vi "endVolume.vi"(8 "error in (no error)":errorcluster, 9 "com queue":refnum<queue>, 10 "scan info":T2, 11 "reader status in":T1) -> (0 "error out":errorcluster, 1 "com queue out":refnum<queue>, 3 "reader status out":T1)   [LabVIEW 2010]
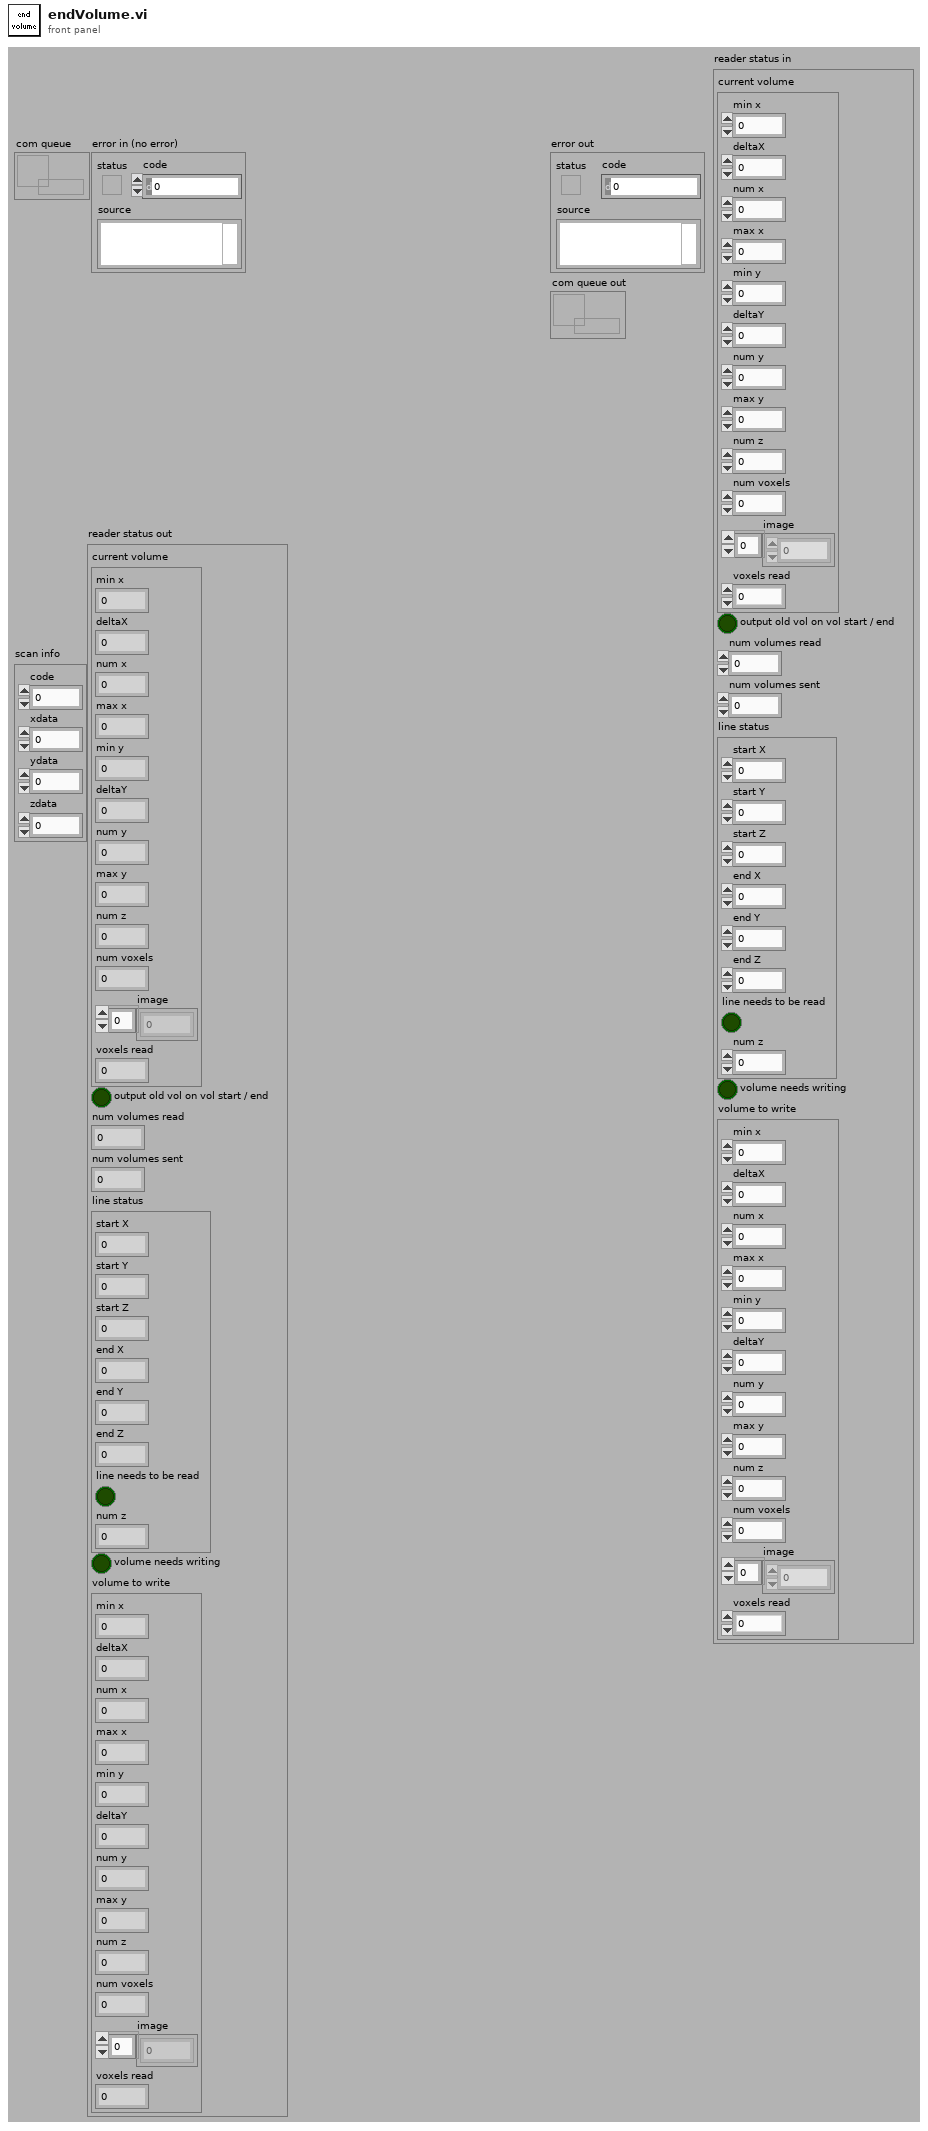
[diagram p1: front panel]
types:
  T1 = cluster{"current volume":cluster{"min x":i16, "deltaX":dbl, "num x":u32, "max x":i16, "min y":i16, "deltaY":dbl, "num y":u32, "max y":i16, "num z":u32, "num voxels":u32, "image":u32[], "voxels read":u32}, "output old vol on vol start / end":bool, "num volumes read":u32, "num volumes sent":u32, "line status":cluster{"start X":i16, "start Y":i16, "start Z":i16, "end X":i16, "end Y":i16, "end Z":i16, "line needs to be read":bool, "num z":u8}, "volume needs writing":bool, "volume to write":cluster{"min x":i16, "deltaX":dbl, "num x":u32, "max x":i16, "min y":i16, "deltaY":dbl, "num y":u32, "max y":i16, "num z":u32, "num voxels":u32, "image":u32[], "voxels read":u32}}
  T2 = cluster{"code":i32, "xdata":i32, "ydata":i32, "zdata":i32}
  T3 = enum16{"NONE", "VOLUME_START", "LINE_START", "LINE_END", "VOLUME_END"}
  T4 = cluster{"min x":i16, "deltaX":dbl, "num x":u32, "max x":i16, "min y":i16, "deltaY":dbl, "num y":u32, "max y":i16, "num z":u32, "num voxels":u32, "image":u32[], "voxels read":u32}
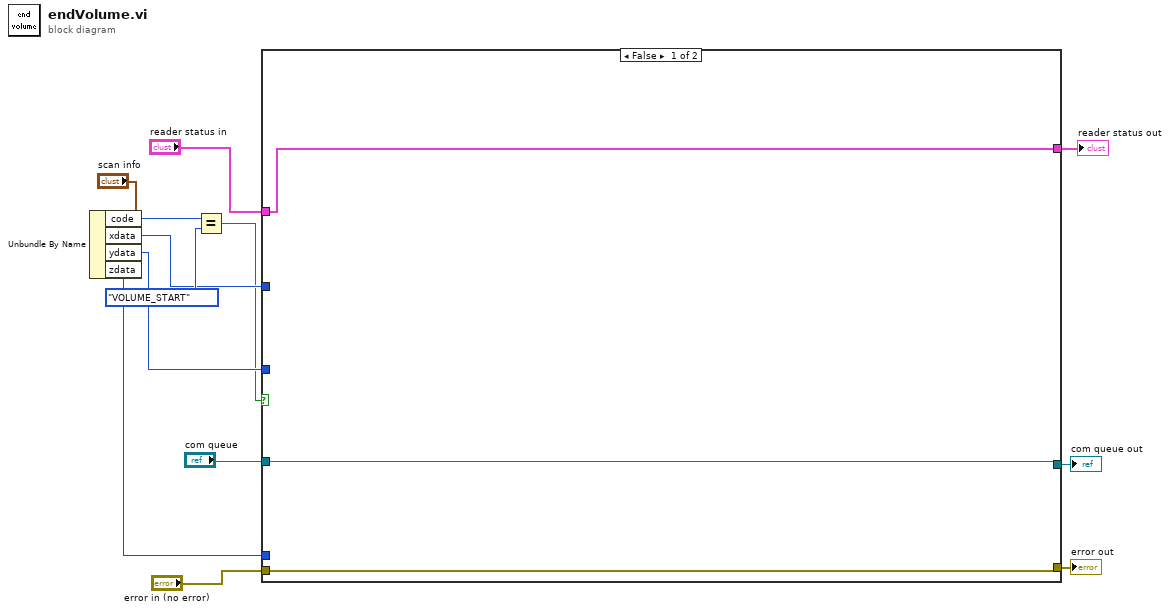
[diagram p0: block diagram]
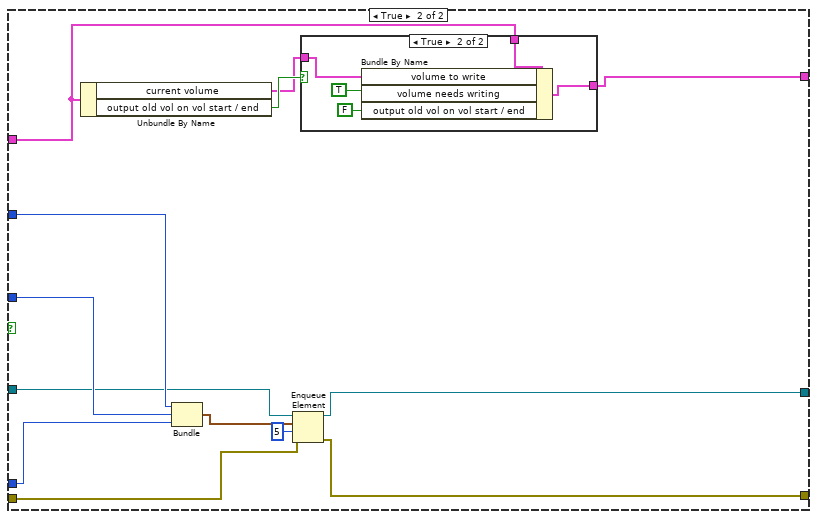
[diagram p2: hidden frame]
diagram:
  n1 = Unbundle By Name("scan info") -> ("code"=w12:i32, "xdata"=w10:i32, "ydata"=w9:i32, "zdata"=w8:i32)
  n2 = Equal?(x=w12, y=T3."VOLUME_START" ("message")) -> (x = y?=w6:bool)
  n3 = case shown="False" w6 {
    tunnel: w10 -> [_ w25]
    tunnel: w9 -> [_ w24]
    tunnel: w8 -> [_ w23]
    tunnel: "reader status in" -> [w16 w27]
    tunnel: [w16 w26] -> w5
    tunnel: "error in (no error)" -> [w15 w21]
    tunnel: [w15 w20] -> w3
    tunnel: "com queue" -> [w14 w18]
    tunnel: [w14 w17] -> w1
    frame False {
    }
    frame True {
      n4 = Unbundle By Name(w27) -> ("current volume"=w28:T4, "output old vol on vol start / end"=w29:bool)
      n5 = Bundle("xdata"=w25, "ydata"=w24, "zdata"=w23) -> (w22:cluster{"xdata":i32, "ydata":i32, "zdata":i32})  [unwired: 1 in]
      n6 = Enqueue Element(queue=w18, element=w22, timeout in ms (-1)=5, error in (no error)=w21) -> (queue out=w17:refnum<queue>, error out=w20:errorcluster)  [unwired: 1 out]
      n7 = case shown="True" w29 {
        tunnel: w28 -> [_ w35]
        tunnel: [w30 w33] -> w26
        tunnel: w27 -> [w30 w32]
        frame False {
        }
        frame True {
          n8 = Bundle By Name(cluster=w32, "volume to write"=w35, "volume needs writing"=TRUE, "output old vol on vol start / end"=FALSE) -> (w33:T1)
        }
      }
    }
  }
  "reader status out" <- w5
  "error out" <- w3
  "com queue out" <- w1
